vi "Do.vi"(8 "error in (no error)":errorcluster, 10 "Actor in":refnum<class "Actor.lvclass">, 11 "Set Length Msg":refnum<class "Set Length Msg.lvclass">) -> (0 "error out":errorcluster, 2 "Actor out":refnum<class "Actor.lvclass">)   [LabVIEW 2021, in "BNT_ULx.lvlib" / "Set Length Msg.lvclass"]
doc: "This VI delivers the message to the actor by calling the appropriate method(s) on the actor."
uses:
  Set Length Msg.lvclass
  <vilib>/ActorFramework/Actor/Actor.lvclass
  C:/Users/Holger/Documents/LVP/BNT/PGC/Packages/CSPP_Core/Messages/CSPP_PVUpdate Msg/CSPP_PVUpdate Msg.lvclass
  BNT_ULx-MCSV-DOPWM/BNT_ULx-MCSV-DOPWM.lvclass
  C:/Program Files (x86)/National Instruments/LabVIEW 2021/vi.lib/ActorFramework/Actor/Actor.lvclass
  CSPP_Core/Messages/CSPP_PVUpdate Msg/CSPP_PVUpdate Msg.lvclass/CSPP_PVUpdate Msg.ctl
  CSPP_Core/Classes/CSPP_ProcessVariables/ProcessVariable/PV.lvclass/PV.ctl
  Set Length Msg.lvclass/Set Length Msg.ctl
  CSPP_Core/Libraries/Utilities/Extract URL Info.vi
  CSPP_Core/Classes/CSPP_ProcessVariables/ProcessVariable/PV.lvclass
  CSPP_Core/Messages/CSPP_PVUpdate Msg/CSPP_PVUpdate Msg.lvclass
  CSPP_Core/Libraries/Utilities/CSPP_Utilities.lvlib
  C:/Users/Holger/Documents/LVP/BNT/PGC/Packages/BNT_ULx/BNT_ULx-MCSV/BNT_ULx-MCSV.lvclass
  C:/Users/Holger/Documents/LVP/BNT/PGC/Packages/CSPP_Core/Actors/CSPP_DeviceActor/CSPP_DeviceActor.lvclass
  C:/Users/Holger/Documents/LVP/BNT/PGC/Packages/CSPP_Core/Actors/CSPP_BaseActor/CSPP_BaseActor.lvclass
  C:/Users/Holger/Documents/LVP/BNT/PGC/Packages/BNT_ULx/BNT_ULx-MCSV-DOPWM/BNT_ULx-MCSV-DOPWM.lvclass
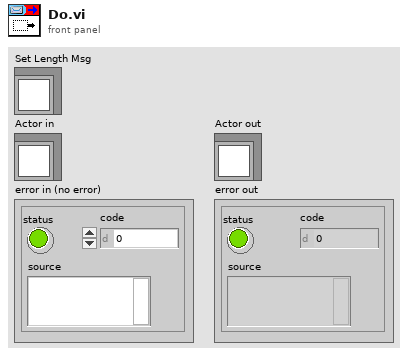
[diagram p1: front panel]
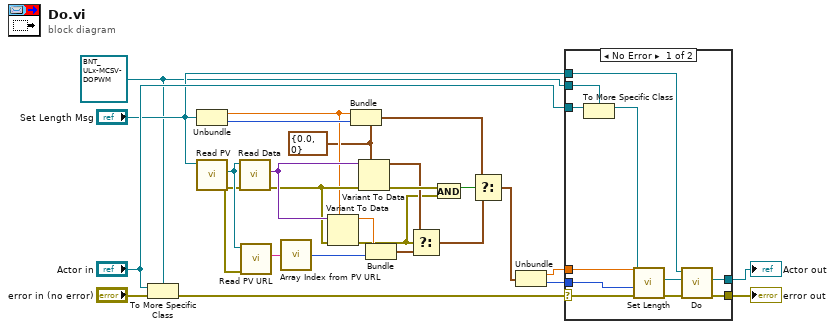
[diagram p0: block diagram]
diagram:
  w3 = refnum<class "BNT_ULx-MCSV-DOPWM.lvclass"> refnum ("BNT_ULx.lvlib:BNT_ULx-MCSV-DOPWM.lvclass")
  w4 = cluster{"PWM Length":dbl[unit], "Line":i32} {"PWM Length"=0.0, "Line"=0} ("cluster")
  n1 = To More Specific Class(target class=w3, reference="Actor in", error in="error in (no error)") -> (error out=w23:errorcluster)  [unwired: 1 out]
  n2 = Unbundle ("Pre-Unbundler")("Set Length Msg") -> (w12:dbl[unit], w18:i32)
  n3 = call "Read PV.vi"("CS++PVUpdate Msg in"="Set Length Msg") -> ("error out"=w15:errorcluster, "PV"=w16:refnum<class "PV.lvclass">)  [unwired: 8 in, 1 out]
  n4 = call "Read Data.vi"("error in (no error)"=w15, "PV in"=w16) -> ("error out"=w13:errorcluster, "Data"=w14:variant)  [unwired: 7 in, 1 out]
  n5 = call "Read PV URL.vi"("error in (no error)"=w15, "PV in"=w16) -> ("PV URL"=w1:string)  [unwired: 7 in, 2 out]
  n6 = call "Array Index from PV URL.vi"("PV-URL"=w1) -> ("Index"=w2:i32)
  n7 = Variant To Data(error in=w13, type=w12, Variant=w14) -> (data=w11:dbl[unit], error out=w7:errorcluster)
  n8 = Bundle ("Pre-Bundler")(cluster=w4, "PWM Length"=w12, "Line"=w18) -> (w19:cluster{"PWM Length":dbl[unit], "Line":i32})
  n9 = Variant To Data(error in=w13, type=w4, Variant=w14) -> (data=w10:cluster{"PWM Length":dbl[unit], "Line":i32}, error out=w20:errorcluster)
  n10 = Bundle ("Pre-Bundler")("PWM Length"=w11, "Index"=w2) -> (w17:cluster{"PWM Length":dbl[unit], "Index":i32})  [unwired: 1 in]
  n11 = Select ("MainSelect")(t=w10, s=w7, f=w17) -> (s? t:f=w9:cluster{"PWM Length":dbl[unit], "Index":i32})
  n12 = And(x=w20, y=w7) -> (x .and. y?=w8:bool)
  n13 = Select ("MainSelect")(t=w19, s=w8, f=w9) -> (s? t:f=w6:cluster{"PWM Length":dbl[unit], "Index":i32})
  n14 = Unbundle ("Main-Unbundler")(w6) -> ("PWM Length"=w22:dbl[unit], "Index"=w21:i32)
  n15 = case shown="No Error" w23 {
    selector: w23 -> [w31 w40]
    tunnel: [w35 w40] -> w26
    tunnel: [w36 w39] -> w25
    tunnel: "Actor in" -> [w38 w39]
    tunnel: w3 -> [w37 _]
    tunnel: "Set Length Msg" -> [w34 _]
    tunnel: w22 -> [w33 _]
    tunnel: w21 -> [w32 _]
    frame No Error {
      n16 = To More Specific Class ("To More Specific Class (internal)")(target class=w37, reference=w38) -> (specific class reference=w30:refnum<class "BNT_ULx-MCSV-DOPWM.lvclass">)  [unwired: 1 in, 1 out]
      n17 = call "Set Length.vi"("error in"=w31, "Line"=w32, "PWM Length"=w33, "BNT_ULx-MCSV-DOPWM in"=w30) -> ("error out"=w28:errorcluster, "BNT_ULx-MCSV-DOPWM out"=w29:refnum<class "BNT_ULx-MCSV-DOPWM.lvclass">)  [unwired: 6 in]
      n18 = call-parent "Do.vi"("error in (no error)"=w28, "Actor in"=w29, "CS++PVUpdate Msg"=w34) -> ("error out"=w35:errorcluster, "Actor out"=w36:refnum<class "Actor.lvclass">)  [unwired: 7 in]
    }
    frame Error {
    }
  }
  "error out" <- w26
  "Actor out" <- w25
